vi "ReadIOPubEvent.vi"(8 "error in (no error)":errorcluster, 11 "object in":refnum<class "JuPyter_Client.lvclass">) -> (0 "error out":errorcluster, 2 "Message Event":refnum<user-event>, 3 "object out":refnum<class "JuPyter_Client.lvclass">)   [LabVIEW 2018, in "JuPyter_Client.lvclass"]
doc: "Either return the existing IOPub event or generate a new one"
uses:
  JuPyter_Client.lvclass
  Base Classes/Message Class/Message Class.lvclass
  JuPyter_Client.lvclass/JuPyter_Client.ctl
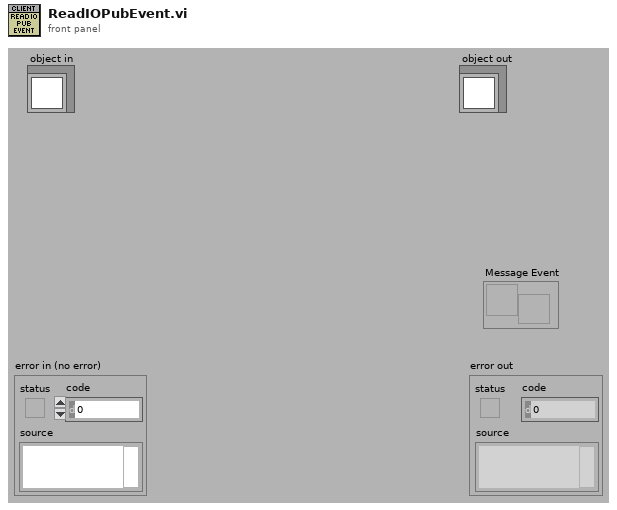
[diagram p1: front panel]
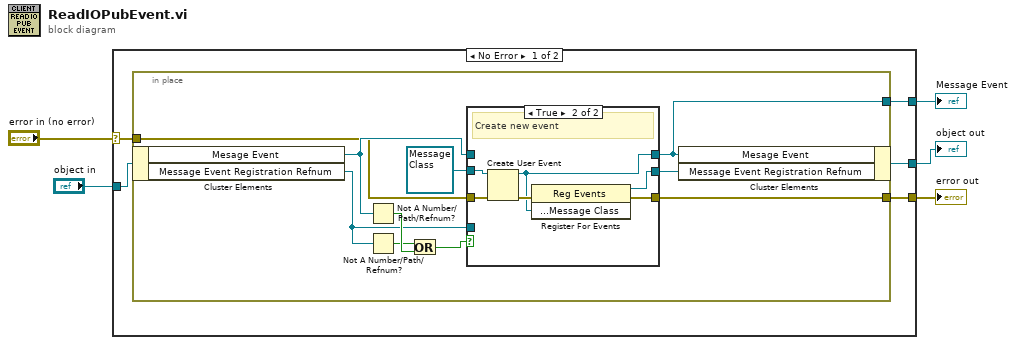
[diagram p0: block diagram]
diagram:
  n1 = case shown="No Error" "error in (no error)" {
    selector: "error in (no error)" -> [w8 w31]
    tunnel: [w7 w31] -> w4
    tunnel: [w6 w30] -> w2
    tunnel: "object in" -> [w9 w30]
    tunnel: [w10 _] -> w1
    frame No Error {
      n2 = in-place {
        in-place-border: [w18] -> w10
        in-place-border: w8 -> [w16]
        in-place-border: [w15] -> w7
        n3 = in-place-cluster #1(w9) -> ("Mesage Event"=w17:refnum<user-event>, "Message Event Registration Refnum"=w13:refnum<event-registration>)
        n4 = Not A Number/Path/Refnum?(number/path/refnum=w17) -> (NaN/Path/Refnum?=w19:bool)
        n5 = Not A Number/Path/Refnum?(number/path/refnum=w13) -> (NaN/Path/Refnum?=w11:bool)
        n6 = Or(x=w11, y=w19) -> (x .or. y?=w12:bool)
        n7 = case shown="True" w12 {
          tunnel: refnum<class "Message Class.lvclass"> refnum ("ClientMessaging.lvlib:Message Class") -> [_ w29]
          tunnel: [w23 w27] -> w18
          tunnel: w17 -> [w23 _]
          tunnel: w16 -> [w22 w26]
          tunnel: [w22 w25] -> w15
          tunnel: [w21 w24] -> w14
          tunnel: w13 -> [w21 _]
          frame False {
            # "Reuse existing event"
          }
          frame True {
            # "Create new event"
            n8 = Create User Event(user event datatype=w29, error in=w26) -> (user event=w27:refnum<user-event>, error out=w28:errorcluster)
            n9 = register-events(error in=w28, w27) -> (reference out=w24:refnum<event-registration>, error out=w25:errorcluster)  [unwired: 1 in]
          }
        }
        n10 = in-place-cluster #1("Mesage Event"=w18, "Message Event Registration Refnum"=w14) -> (w6:refnum<class "JuPyter_Client.lvclass">)
      }
    }
    frame Error {
    }
  }
  "error out" <- w4
  "object out" <- w2
  "Message Event" <- w1
